vi "_emi_ SMLoop start condition.vi"(0 "Loop ID in":u16, 11 "error in (no error)":errorcluster) -> (4 "Loop ID out":u16, 13 "Klar til start":bool, 15 "error out":errorcluster)   [LabVIEW 2011]
doc: "Check wheter a loop should start. based on loop enable(Loop control),\n\nExecutes as normal on error"
uses:
  Loop control/Private/_emi_Loop control int action.ctl
  _emi_ SMLoop restart type.ctl
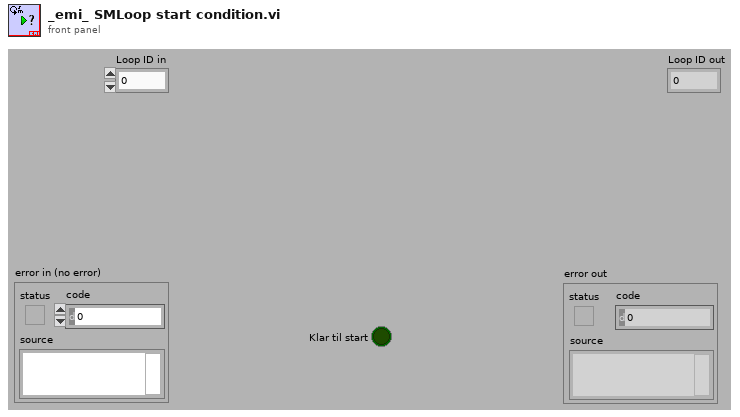
[diagram p1: front panel]
types:
  T1 = typedef "_emi_Loop control int action.ctl" = enum16{"Init index", "Get index", "Set index", "Get Size"}
  T2 = typedef "_emi_ SMLoop restart type.ctl" = enum16{"Normal", "Stop", "Stopped"}
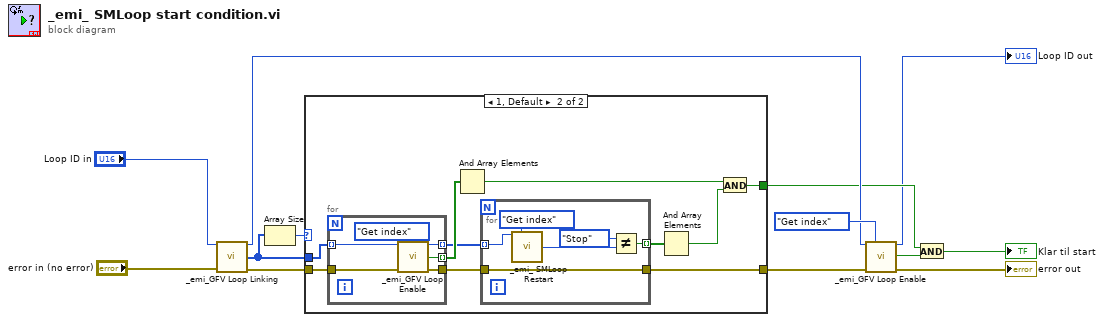
[diagram p0: block diagram]
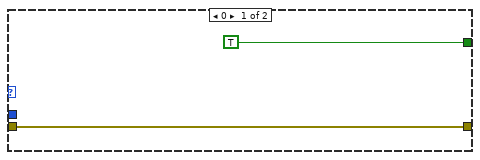
[diagram p2: hidden frame]
diagram:
  n1 = call "_emi_GFV Loop Linking.vi"("Loop Index/Numb"="Loop ID in", "error in (no error)"="error in (no error)") -> ("Index out"=w11:u16, "Linked indexes out"=w8:u16[], "error out"=w9:errorcluster)  [unwired: 10 in, 1 out]
  n2 = Array Size(array=w8) -> (size(s)=w10:i32)
  n3 = case shown="1, Default" w10 {
    tunnel: w9 -> [w14 w25]
    tunnel: w8 -> [_ w22]
    tunnel: [w14 w21] -> w6
    tunnel: [TRUE w17] -> w7
    frame 0 {
    }
    frame 1, Default {
      n4 = for {
        tunnel: w25 -> [w37]
        tunnel: [w36] -> w20
        tunnel: [w34] -> w24 mode=indexing
        tunnel: w22 -> [w33] mode=indexing
        tunnel: [w32] -> w19 mode=indexing
        n5 = call "_emi_GFV Loop Enable.vi"("Loop Index/Numb"=w33, "Action(Get Index)"=_emi_Loop_control_int_action."Get index", "error in (no error)"=w37) -> ("Index out"=w32:u16, "Loop Enable Out"=w34:bool, "error out"=w36:errorcluster)  [unwired: 9 in, 1 out]
      }
      n6 = And Array Elements(Boolean array=w24) -> (logical AND=w23:bool)
      n7 = for {
        tunnel: w20 -> [w31]
        tunnel: [w31] -> w21
        tunnel: w19 -> [w30] mode=indexing
        tunnel: [w26] -> w18 mode=indexing
        n8 = call "_emi_ SMLoop Restart.vi"("Loop Index/Numb"=w30, "Action(Get Index)"=_emi_Loop_control_int_action."Get index") -> ("Value out"=w28:T2)  [unwired: 11 in, 2 out]
        n9 = Not Equal?(x=_emi__SMLoop_restart_type."Stop", y=w28) -> (x != y?=w26:bool)
      }
      n10 = And Array Elements(Boolean array=w18) -> (logical AND=w16:bool)
      n11 = And(x=w23, y=w16) -> (x .and. y?=w17:bool)
    }
  }
  n12 = call "_emi_GFV Loop Enable.vi"("Loop Index/Numb"=w11, "Action(Get Index)"=_emi_Loop_control_int_action."Get index", "error in (no error)"=w6) -> ("Index out"=→"Loop ID out":u16, "Loop Enable Out"=w12:bool, "error out"=→"error out":errorcluster)  [unwired: 9 in, 1 out]
  n13 = And(x=w7, y=w12) -> (x .and. y?=→"Klar til start":bool)
